vi "Mark Favorite.vi"(8 "error in (no error)":errorcluster, 10 "Favorite?":bool, 11 "ID":u32) -> (0 "error out":errorcluster, 3 "dup ID":u32)   [LabVIEW 2014, in "Map Data.lvlib"]
doc: "Marks or unmarks a single contact as being a favorite in the address book data store."
uses:
  Map Data.lvlib
  MapDatas.ctl
  MapCommand.ctl
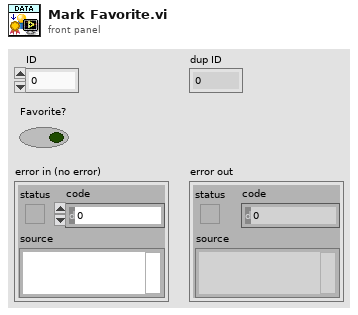
[diagram p1: front panel]
types:
  T1 = typedef "Map Data.lvlib/MapCommand.ctl" = enum16{"Load", "Update Cursor", "Save", "Get All Data", "Get Single Data", "Set Single Data", "Delete All", "Remove Single Data", "Set Favorite Status", "Is Data Modified", "Import Data"}
  T2 = typedef "Map Data.lvlib/MapDatas.ctl" = cluster{"X":dbl, "Y":dbl, "Z":dbl, "heading":dbl, "X2":dbl, "Y2":dbl, "Z2":dbl}
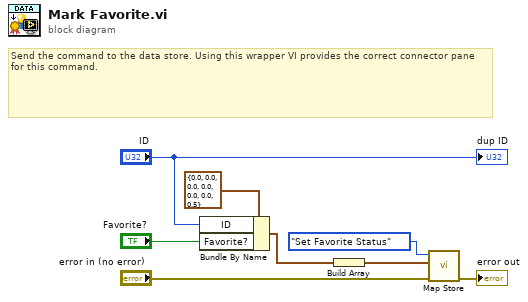
[diagram p0: block diagram]
diagram:
  # "Send the command to the data store. Using this wrapper VI provides the correct connector pane for this command."
  n1 = Bundle By Name(cluster=T2 {"X"=0.0, "Y"=0.0, "Z"=0.0, "heading"=0.0, "X2"=0.0, "Y2"=0.0, "Z2"=0.5} ("Contact"), "ID"="ID", "Favorite?"="Favorite?") -> (w6:T2)
  n2 = Build Array(w6) -> (w1:T2[])
  n3 = call "Map Store.vi"("error in (no error)"="error in (no error)", "All Lines"=w1, "Command"=MapCommand."Set Favorite Status") -> ("error out"=→"error out":errorcluster)  [unwired: 5 in, 3 out]
  "dup ID" <- "ID"
